vi "FINS out-setup.vi"(8 "error i":errorcluster, 10 "SA1":u8) -> (0 "error o":errorcluster, 2 "msg":string, 3 "FINS Header":T1 {"SNA" max=127 format="%x"; "SA2" max=254 step=1 format="%x"; "SA1" format="%x"; "DA2" max=254 step=1 format="%x"; "DA1" format="%x"; "DNA" max=127 step=1 format="%x"})   [LabVIEW 2020]
uses:
  FINS/FINS_header.ctl
  FINS/FINS CMD item.ctl
  FINS/FINS TCP.lvlib
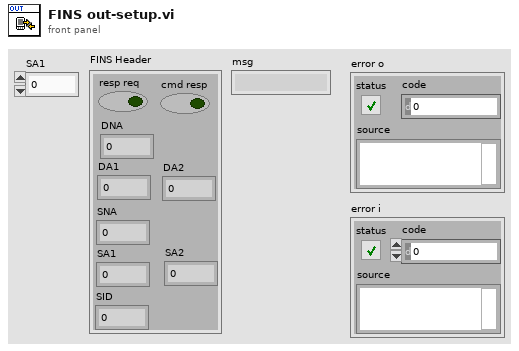
[diagram p1: front panel]
types:
  T1 = typedef "FINS TCP.lvlib/FINS_header.ctl" = cluster{"resp req":bool, "cmd resp":bool, "SID":u8, "DNA":u8, "DA1":u8, "DA2":u8, "SA1":u8, "SA2":u8, "SNA":u8}
  T2 = typedef "FINS TCP.lvlib/FINS CMD item.ctl" = enum16{"FINS_UNKNOWN", "FINS_SETUP", "MEMORY AREA READ", "MEMORY AREA WRITE", "MEMORY AREA FILL", "MULTIPLE MEMORY AREA READ", "MEMORY AREA TRANSFER", "PARAMETER AREA READ", "PARAMETER AREA WRITE", "PARAMETER AREA CLEAR", "PROGRAM AREA PROTECT", "PROGRAM AREA PROTECT CLEAR", "PROGRAM AREA READ", "PROGRAM AREA WRITE", "PROGRAM AREA CLEAR", "RUN", "STOP", "CONTROLLER DATA READ", "CONNECTION DATA READ", "CONTROLLER STATUS READ", "CYCLE TIME READ", "CLOCK READ", "CLOCK WRITE", "MESSAGE READ", "MESSAGE CLEAR", "FAL/FALS READ", "ACCESS RIGHT ACQUIRE", "ACCESS RIGHT FORCED ACQUIRE", "ACCESS RIGHT RELEASE", "ERROR CLEAR", "ERROR LOG READ", "ERROR LOG CLEAR", "FILE NAME READ", "SINGLE FILE READ", "SINGLE FILE WRITE", "MEMORY CARD FORMAT", "FILE DELETE", "VOLUME LABEL CREATE/DELETE", "FILE COPY", "FILE NAME CHANGE", "FILE DATA CHECK", "MEMORY AREA FILE TRANSFER", "PARAMETER AREA FILE TRANSFER", "PROGRAM AREA FILE TRANSFER", "FORCED SET/RESET", "FORCED SET/RESET CANCEL"}
  T3 = typedef "FINS TCP.lvlib/FINS CMD.ctl" = cluster{"MR":u8, "SR":u8, "name":string}
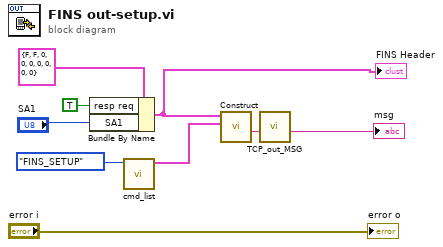
[diagram p0: block diagram]
diagram:
  n1 = Bundle By Name(cluster=T1 {"resp req"=FALSE, "cmd resp"=FALSE, "SID"=0, "DNA"=0, "DA1"=0, "DA2"=0, "SA1"=0, "SA2"=0, "SNA"=0} ("FINS Header"), "resp req"=TRUE, "SA1"="SA1") -> (w3:T1)
  "FINS Header" <- w3
  n2 = call "cmd_list.vi"("CMD"=FINS_CMD_item."FINS_SETUP") -> ("cmd"=w7:T3)  [unwired: 9 in, 1 out]
  n3 = call "Construct.vi"("FINS CMD"=w7, "FINS Header"=w3) -> ("msg"=w9:string)  [unwired: 9 in]
  n4 = call "TCP_out_MSG.vi"("msgin"=w9) -> ("msg"=→"msg":string)  [unwired: 10 in]
  "error o" <- "error i"
